vi "Reverse 2D Array (U16)__ogtk.vi"(2 "by rows or columns (rows)":enum16{"rows", "columns"}(ring), 3 "Array":u16[][](array[numeric])) -> (1 "Reversed Array":u16[][](array[numeric]))   [LabVIEW 2020]
doc: "This polymorphic VI reverses the input 2D <B>Array</B> and outputs the result as <B>Reversed Array</B>. Use the <B>by rows or columns</B> input to specify whether to sort by row or by column."
panel:
  # "Reverse 2D Array.vi\n\nThis VI reverses, by row or by column, 2D array of any size.\n\nPlease visit http://www.OpenG.org to learn about the\nOpen Source LabVIEW software movement.\n\nNOTICE -- YOU MUST LEAVE THIS NOTICE IN PLACE.  PER THE TERMS OF THE LICENSE BELOW, YOU MAY SUBLICENSE THIS SOFTWARE \nIN ANY WAY THAT DOES NOT CONFLICT WITH THIS LICENSE.\n\n### BSD License (http://www.opensource.org/licenses/bsd-license.php) Begin ###\n \nCopyright (c) 2002, Jim Kring <jim@jimkring.com>\nCopyright (c) 2002, Cal-Bay Systems, Inc. <info@calbay.com>\n\nAll rights reserved.\n\nRedistribution and use in source and binary forms, with or without modification, are permitted provided that the following conditions are met:\n\n    * Redistributions of source code must retain the above copyright notice, this list of conditions and the following disclaimer.\n    * Redistributions in binary form must reproduce the above copyright notice, this list of conditions and the following disclaimer in the \n       documentation and/or other materials provided with the distribution.\n    * Neither the name of SciWare, James Kring, Inc., nor the names of its contributors may be used to endorse or promote products derived \n       from this software without specific prior written permission.\n\nTHIS SOFTWARE IS PROVIDED BY THE COPYRIGHT HOLDERS AND CONTRIBUTORS \"AS IS\" AND ANY EXPRESS OR IMPLIED WARRANTIES, \nINCLUDING, BUT NOT LIMITED TO, THE IMPLIED WARRANTIES OF MERCHANTABILITY AND FITNESS FOR A PARTICULAR PURPOSE ARE \nDISCLAIMED. IN NO EVENT SHALL THE COPYRIGHT OWNER OR CONTRIBUTORS BE LIABLE FOR ANY DIRECT, INDIRECT, INCIDENTAL,\n SPECIAL, EXEMPLARY, OR CONSEQUENTIAL DAMAGES (INCLUDING, BUT NOT LIMITED TO, PROCUREMENT OF SUBSTITUTE GOODS OR \nSERVICES; LOSS OF USE, DATA, OR PROFITS; OR BUSINESS INTERRUPTION) HOWEVER CAUSED AND ON ANY THEORY OF LIABILITY, \nWHETHER IN CONTRACT, STRICT LIABILITY, OR TORT (INCLUDING NEGLIGENCE OR OTHERWISE) ARISING IN ANY WAY OUT OF THE USE \nOF THIS SOFTWARE, EVEN IF ADVISED OF THE POSSIBILITY OF SUCH DAMAGE.\n\n### BSD License End ###"
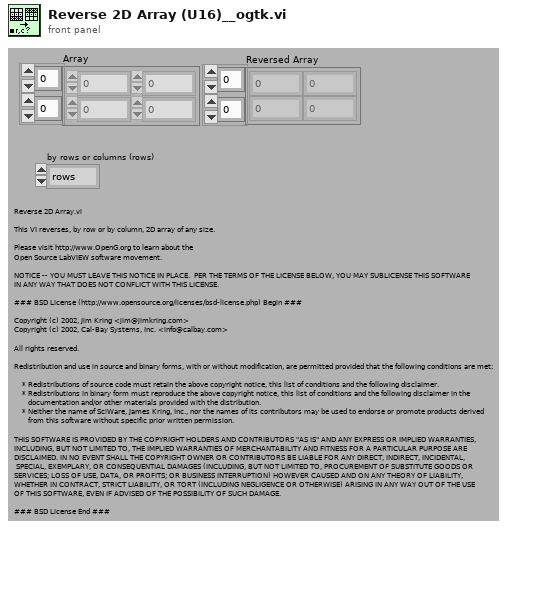
[diagram p1: front panel]
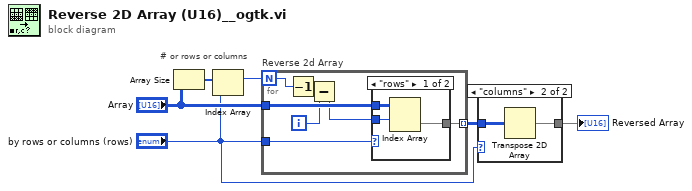
[diagram p0: block diagram]
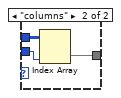
[diagram p3: hidden frame]
diagram:
  # "# or rows or columns"
  n1 = Array Size(array="Array") -> (size(s)=w5:i32[])
  n2 = Index Array(array=w5, index="by rows or columns (rows)") -> (element=w4:i32)
  n3 = for "Reverse 2d Array" {
    N: w4 -> [w12]
    tunnel: "Array" -> [w13]
    tunnel: [w8] -> w2 mode=indexing
    tunnel: "by rows or columns (rows)" -> [w7]
    i -> [w10]
    n4 = Decrement(x=w12) -> (x-1=w11:i32)
    n5 = Subtract(x=w11, y=w10) -> (x-y=w9:i32)
    n6 = case shown="\"rows\"" w7 {
      tunnel: w13 -> [w16 w19]
      tunnel: w9 -> [w15 w17]
      tunnel: [w14 w18] -> w8
      frame "rows" {
        n7 = Index Array(array=w16, index (row)=w15) -> (element=w14:u16[])  [unwired: 1 in]
      }
      frame "columns" {
        n8 = Index Array(array=w19, index (col)=w17) -> (element=w18:u16[])  [unwired: 1 in]
      }
    }
  }
  n9 = case shown="\"columns\"" "by rows or columns (rows)" {
    tunnel: w2 -> [w20 w22]
    tunnel: [w20 w21] -> w1
    frame "rows" {
    }
    frame "columns" {
      n10 = Transpose 2D Array(2D array=w22) -> (transposed array=w21:u16[][])
    }
  }
  "Reversed Array" <- w1
